vi "Ctor.vi"(8 "error in (no error)":errorcluster) -> (0 "error out":errorcluster, 3 "PathTree out":refnum<class "PathTree.lvclass">)   [LabVIEW 2020, in "PathTree.lvlib" / "PathTree.lvclass"]
uses:
  PathTree.lvclass
  Ref Data.ctl
  PathTree.lvclass/PathTree.ctl
  PathTreeNode/PathTreeNode.lvclass
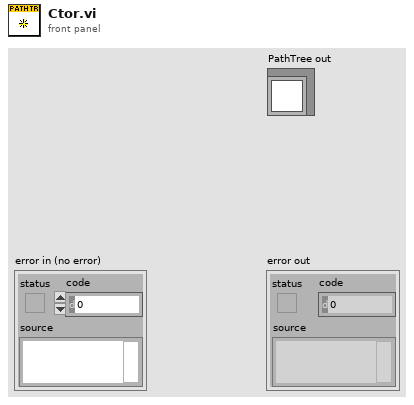
[diagram p1: front panel]
types:
  T1 = typedef "PathTree.lvlib/PathTree.lvclass/Ref Data.ctl" = cluster{"Root":refnum<class>}
  T2 = typedef "Advanced Structures.lvlib/PathTree.lvclass/Ref Data.ctl" = cluster{"Root":refnum<class>}
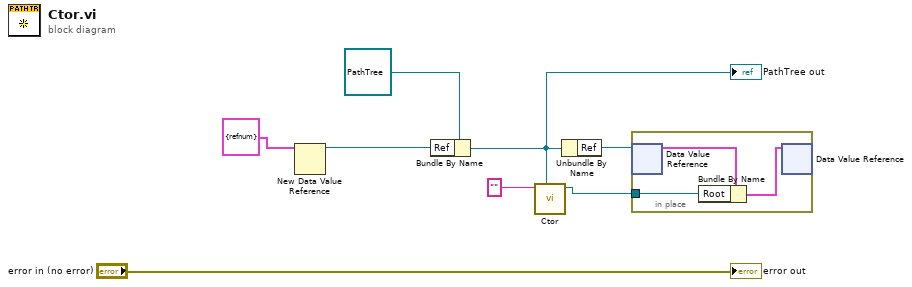
[diagram p0: block diagram]
diagram:
  n1 = New Data Value Reference(data value=T1 {"Root"=refnum} ("Ref Data")) -> (data value reference=w5:refnum<data-value>)  [unwired: 1 in, 1 out]
  n2 = Bundle By Name(cluster=refnum<class "PathTree.lvclass"> refnum ("PathTree in"), "Ref"=w5) -> (w2:refnum<class "PathTree.lvclass">)
  "PathTree out" <- w2
  n3 = call "Ctor.vi"("Tree"=w2, "Token"="") -> ("PathTreeNode out"=w1:refnum<class "PathTreeNode.lvclass">)  [unwired: 8 in, 1 out]
  n4 = Unbundle By Name(w2) -> ("Ref"=w3:refnum<data-value>)
  n5 = in-place {
    in-place-border: w1 -> [w9]
    n6 = in-place-dvr #1(w3) -> (w11:T2)  [unwired: 1 out]
    n7 = Bundle By Name(cluster=w11, "Root"=w9) -> (w10:T2)
    n8 = in-place-dvr #1(w10) -> ()  [unwired: 2 out]
  }
  "error out" <- "error in (no error)"
